vi "create_files_from_dataclust.vi"(8 "error in":errorcluster, 10 "base path":path, 11 "cluster in":variant) -> (0 "error out":errorcluster, 3 "Refnums":refnum<file>[](array[refnum]))   [LabVIEW 2015]
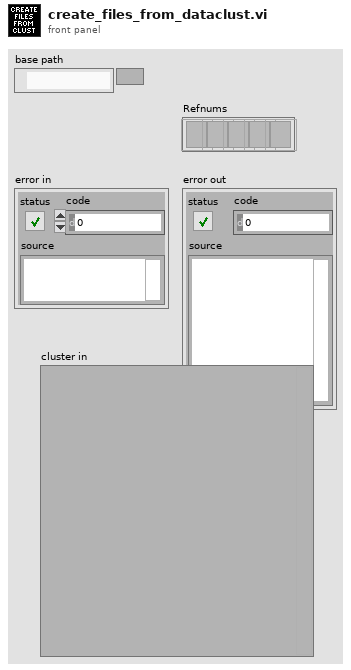
[diagram p1: front panel]
types:
  T1 = enum16{"open", "replace", "create", "open or create", "replace or create", "replace or create with confirmation"}
  T2 = typedef "Type Descriptor Enumeration__ogtk.ctl" = enum8{"<Null>", "I8", "I16", "I32", "I64", "U8", "U16", "U32", "U64", "SGL", "DBL", "EXT", "CSG", "CDB", "CXT", "0x0F", "0x10", "0x11", "0x12", "0x13", "0x14", "Enum U8", "Enum U16", "Enum U32", "Enum U64", "SGL PQ", "DBL PQ", "EXT PQ", "CSG PQ", "CDB PQ", "CXT PQ", "0x1F", "0x20", "Boolean", "0x22", "0x23", "0x24", "0x25", "0x26", "0x27", "0x28", "0x29", "0x2A", "0x2B", "0x2C", "0x2D", "0x2E", "0x2F", "String", "0x31", "Path", "Pict", "0x34", "0x35", "0x36", "DAQ", "0x38", "0x39", "0x3A", "0x3B", "0x3C", "0x3D", "0x3E", "0x3F", "Array", "0x41", "0x42", "0x43", "0x44", "0x45", "0x46", "0x47", "0x48", "0x49", "0x4A", "0x4B", "0x4C", "0x4D", "0x4E", "0x4F", "Cluster", "0x51", "0x52", "Variant", "Waveform", "0x55", "0x56", "0x57", "0x58", "0x59", "0x5A", "0x5B", "0x5C", "0x5D", "0x5E", "0x5F", "0x60", "0x61", "0x62", "0x63", "0x64", "0x65", "0x66", "0x67", "0x68", "0x69", "0x6A", "0x6B", "0x6C", "0x6D", "0x6E", "0x6F", "Refnum"}
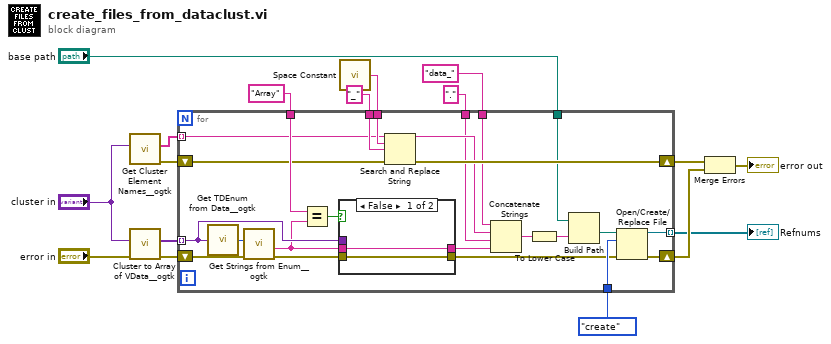
[diagram p0: block diagram]
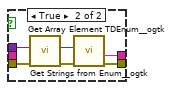
[diagram p2: hidden frame]
diagram:
  n1 = call <userlib>:"Get Cluster Element Names__ogtk.vi"("Cluster"="cluster in") -> ("error out"=w15:errorcluster, "Element Names"=w16:string[])  [unwired: 9 in]
  n2 = call <userlib>:"Cluster to Array of VData__ogtk.vi"("error in (no error)"="error in", "Cluster"="cluster in") -> ("error out"=w14:errorcluster, "Array of VData"=w17:variant[])  [unwired: 8 in]
  n3 = call <vilib>:"Space Constant.vi"() -> ("String"=w13:string)
  n4 = for {
    tunnel: w17 -> [w27] mode=indexing
    tunnel: w16 -> [w18] mode=indexing
    shift-right: [w41] -> w11
    shift-left: w15 -> [w19]
    shift-right: [w34] -> w10
    shift-left: w14 -> [w31]
    tunnel: w13 -> [w39]
    tunnel: "_" ("replace string (\"\")") -> [w38]
    tunnel: "base path" -> [w36]
    tunnel: [w35] -> w9 mode=indexing
    tunnel: T1."create" ("operation (0:open)") -> [w33]
    tunnel: "data_" -> [w26]
    tunnel: "Array" ("x") -> [w25]
    tunnel: "." ("string") -> [w24]
    n5 = call <userlib>:"Get TDEnum from Data__ogtk.vi"("Data"=w27) -> ("Type Descriptor Enumeration"=w32:T2)  [unwired: 4 in]
    n6 = call <userlib>:"Get Strings from Enum__ogtk.vi"("error in (no error)"=w31, "Enum"=w32) -> ("error out"=w29:errorcluster, "String Value"=w23:string)  [unwired: 6 in, 2 out]
    n7 = Equal?(x=w25, y=w23) -> (x = y?=w30:bool)
    n8 = case shown="False" w30 {
      tunnel: w29 -> [w43 w49]
      tunnel: w23 -> [w42 _]
      tunnel: [w43 w46] -> w28
      tunnel: [w42 w45] -> w22
      tunnel: w27 -> [_ w44]
      frame False {
      }
      frame True {
        n9 = call <userlib>:"Get Array Element TDEnum__ogtk.vi"("error in (no error)"=w49, "Array"=w44) -> ("error out"=w47:errorcluster, "Element Type"=w48:T2)  [unwired: 8 in]
        n10 = call <userlib>:"Get Strings from Enum__ogtk.vi"("error in (no error)"=w47, "Enum"=w48) -> ("error out"=w46:errorcluster, "String Value"=w45:string)  [unwired: 6 in, 2 out]
      }
    }
    n11 = Search and Replace String(input string=w18, search string=w39, replace string=w38, error in=w19) -> (result string=w40:string, error out=w41:errorcluster)  [unwired: 4 in, 2 out]
    n12 = Concatenate Strings(w26, w40, w24, w22) -> (w21:string)
    n13 = To Lower Case(string=w21) -> (all lower case string=w20:string)
    n14 = Build Path(base path=w36, name or relative path=w20) -> (appended path=w37:path)
    n15 = Open/Create/Replace File(file path (use dialog)=w37, error in=w28, operation (0:open)=w33) -> (refnum out=w35:refnum<file>, error out=w34:errorcluster)  [unwired: 3 in, 1 out]
  }
  "Refnums" <- w9
  n16 = Merge Errors(w11, w10) -> (→"error out":errorcluster)
